vi "Build Windows Log Path.vi"(7 "Extension":string="csv", 8 "error in (no error)":errorcluster, 9 "Timestamp":bool, 10 "Name":string, 11 "Log File Directory":string) -> (0 "error out":errorcluster, 3 "Log File Path":string)   [LabVIEW 2020]
uses:
  <vilib>/regexp/Match Regular Expression.xnode
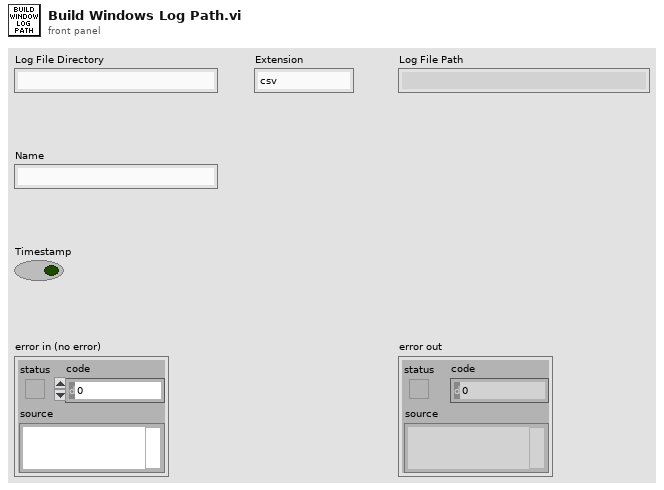
[diagram p1: front panel]
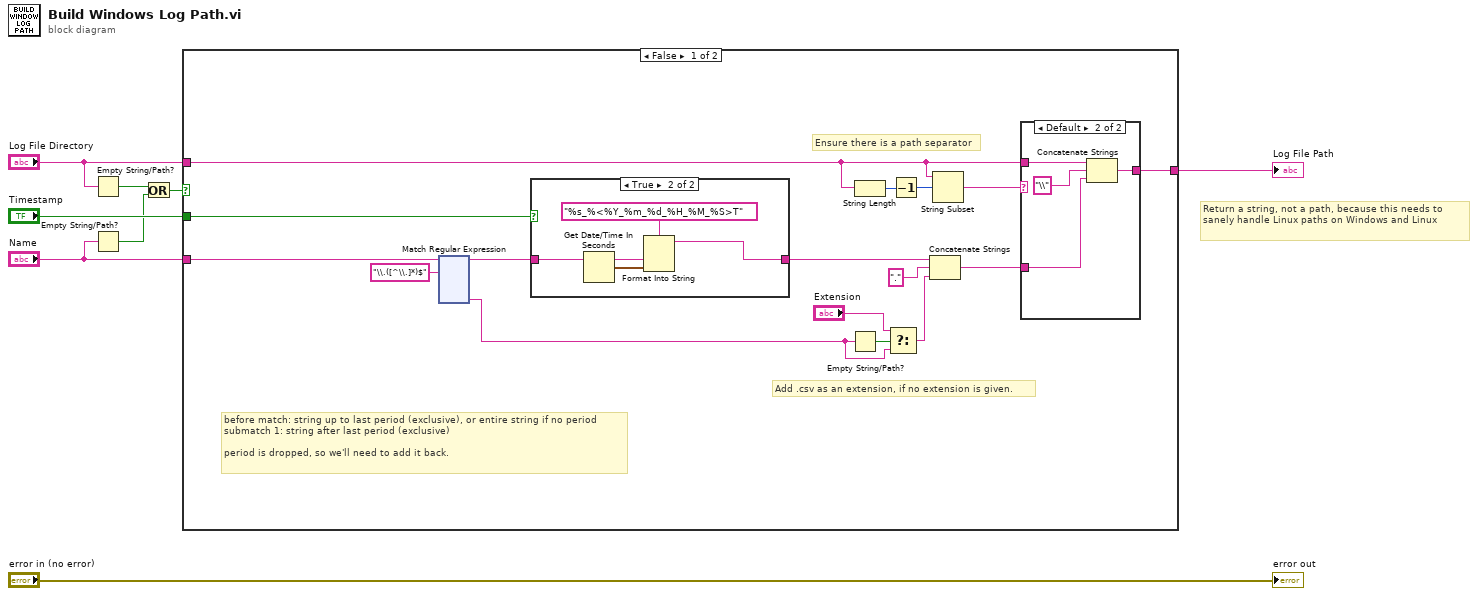
[diagram p0: block diagram]
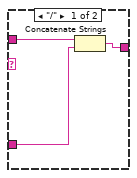
[diagram p2: hidden frame]
diagram:
  # "Return a string, not a path, because this needs to  sanely handle Linux paths on Windows and Linux"
  n1 = Empty String/Path?(string/path="Log File Directory") -> (empty?=w3:bool)
  n2 = Empty String/Path?(string/path="Name") -> (empty?=w2:bool)
  n3 = Or(x=w3, y=w2) -> (x .or. y?=w1:bool)
  n4 = case shown="False" w1 {
    tunnel: "Timestamp" -> [w21 _]
    tunnel: "Log File Directory" -> [w19 _]
    tunnel: [w16 _] -> w6
    tunnel: "Name" -> [w15 _]
    frame False {
      # "Add .csv as an extension, if no extension is given."
      # "Ensure there is a path separator"
      # "before match: string up to last period (exclusive), or entire string if no period\nsubmatch 1: string after last period (exclusive)\n\nperiod is dropped, so we'll need to add it back."
      n5 = xnode "Match Regular Expression"("input string"=w15, "regular expression"="\\.([^\\.]*)$") -> ("before match"=w13:string, "submatch 1"=w9:string)  [unwired: 4 in, 4 out]
      n6 = case shown="True" w21 {
        tunnel: w13 -> [w148 w152]
        tunnel: [w148 w151] -> w22
        frame False {
        }
        frame True {
          n7 = Get Date/Time In Seconds() -> (seconds since 1Jan1904=w149:timestamp)
          n8 = Format Into String(format string="%s_%<%Y_%m_%d_%H_%M_%S>T", w152, w149) -> (resulting string=w151:string)  [unwired: 2 in, 1 out]
        }
      }
      n9 = Empty String/Path?(string/path=w9) -> (empty?=w12:bool)
      n10 = String Length(string=w19) -> (length=w20:i32)
      n11 = Select(t="Extension", s=w12, f=w9) -> (s? t:f=w10:string)
      n12 = Decrement(x=w20) -> (x-1=w18:i32)
      n13 = Concatenate Strings(w22, "." ("string"), w10) -> (w24:string)
      n14 = String Subset(string=w19, offset (0)=w18) -> (substring=w17:string)  [unwired: 1 in]
      n15 = case shown="Default" w17 {
        tunnel: w24 -> [w143 w147]
        tunnel: w19 -> [w142 w146]
        tunnel: [w141 w144] -> w16
        frame "/" {
          n16 = Concatenate Strings(w142, w143) -> (w141:string)
        }
        frame Default {
          n17 = Concatenate Strings(w146, "\\" ("string"), w147) -> (w144:string)
        }
      }
    }
    frame True {
    }
  }
  "Log File Path" <- w6
  "error out" <- "error in (no error)"
